vi "Host Key.vi"(7 "Address":string, 8 "Error In":errorcluster) -> (0 "Error Out":errorcluster)   [LabVIEW 2018, in "Tests.lvlib" / "Session.lvlib"]
uses:
  Session.lvlib
  src/Toolkit/API/Session/API/Typedefs/Host Key Types.ctl
  <vilib>/addons/_JKI Toolkits/Caraya/classes/Test/Test.lvclass
  src/Toolkit/API/SSH/SSH.lvclass
  src/Toolkit/API/Session/Session.lvclass
  <vilib>/addons/_JKI Toolkits/Caraya/classes/Assert/Assert.lvclass
  Tests.lvlib
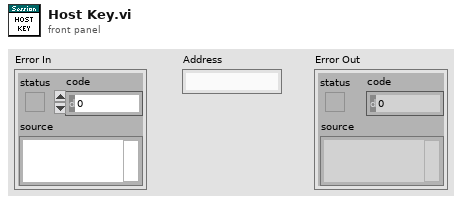
[diagram p1: front panel]
types:
  T1 = typedef "Toolkit.lvlib/Session.lvclass/Host Key Types.ctl" = enum16{"RSA", "DSS", "Unknown"}
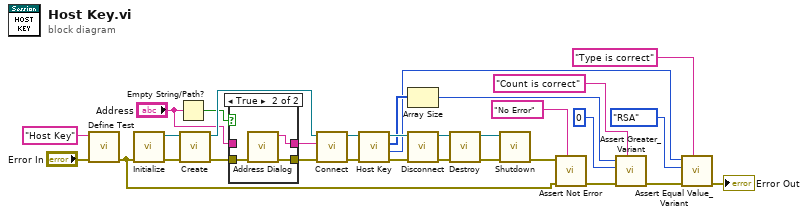
[diagram p0: block diagram]
diagram:
  n1 = call <vilib>:"Define Test.vi"("error in (no error)"="Error In", "Label (VI Title)"="Host Key") -> ("error out"=w26:errorcluster)  [unwired: 9 in]
  n2 = call "Initialize.vi"("Error In"=w26) -> ("Error Out"=w29:errorcluster, "SSH"=w17:refnum<class "SSH.lvclass">)  [unwired: 9 in]
  n3 = Empty String/Path?(string/path="Address") -> (empty?=w22:bool)
  n4 = call "Create.vi"("Error In"=w29, "SSH"=w17) -> ("Error Out"=w20:errorcluster, "Sesssion"=w25:refnum<class "Session.lvclass">)  [unwired: 8 in]
  n5 = case shown="True" w22 {
    tunnel: w20 -> [w32 w36]
    tunnel: [w32 w35] -> w19
    tunnel: [w33 w34] -> w13
    tunnel: "Address" -> [w33 _]
    frame False {
    }
    frame True {
      n6 = call "Address Dialog.vi"("Error In"=w36) -> ("Error Out"=w35:errorcluster, "Address Out"=w34:string)  [unwired: 9 in]
    }
  }
  n7 = call "Connect.vi"("Error In"=w19, "Address"=w13, "Session In"=w25) -> ("Error Out"=w10:errorcluster, "Sesssion Out"=w12:refnum<class "Session.lvclass">)  [unwired: 7 in]
  n8 = call "Host Key.vi"("Error In"=w10, "Session In"=w12) -> ("Error Out"=w9:errorcluster, "Type"=w2:T1, "Host Key"=w8:u8[], "Sesssion Out"=w11:refnum<class "Session.lvclass">)  [unwired: 6 in]
  n9 = Array Size(array=w8) -> (size(s)=w7:i32)
  n10 = call "Disconnect.vi"("Error In"=w9, "Session In"=w11) -> ("Error Out"=w23:errorcluster, "Sesssion Out"=w24:refnum<class "Session.lvclass">)  [unwired: 8 in]
  n11 = call "Destroy.vi"("Error In"=w23, "Session"=w24) -> ("Error Out"=w15:errorcluster, "SSH"=w14:refnum<class "SSH.lvclass">)  [unwired: 8 in]
  n12 = call "Shutdown.vi"("Error In"=w15, "SSH"=w14) -> ("Error Out"=w28:errorcluster)  [unwired: 9 in]
  n13 = call <vilib>:"Assert Not Error.vi"("Label"="No Error", "error in (no error)"=w26, "Not Error?"=w28) -> ("error out"=w18:errorcluster)  [unwired: 8 in]
  n14 = call <vilib>:"Assert Greater_Variant.vi"("Label"="Count is correct", "error in (no error)"=w18, "Y"=0 ("size(s)"), "X"=w7) -> ("error out"=w5:errorcluster)  [unwired: 7 in]
  n15 = call <vilib>:"Assert Equal Value_Variant.vi"("Label"="Type is correct", "error in (no error)"=w5, "Y"=Host_Key_Types."RSA" ("Type"), "X"=w2) -> ("error out"=→"Error Out":errorcluster)  [unwired: 7 in]
